vi "vission comm test.vi"() -> ()   [LabVIEW 2009]
uses:
  vision decoder state typedef.ctl
  behaviors/driveable path/drivable paths global.vi
  behaviors/line driveable paths global.vi
  <vilib>/rvi/DataTransferAndStorage/Container/XNode/niFpgaContainer.xnode
  <vilib>/rvi/FIFO/Fifo_Resource/nirvififoUniquifyingName.vi
panel:
  out "x data":i16
  out "y data":i16
  out "DMA timeout":bool
  out "driveable path lengths":u16[](array[numeric])
  out "decoder state":T1
  out "scan number":u8
  in  "allowed proximity squared":i16=100
  in  "Invert Polarity?":bool
  out "driveable path lengths (lines)":u16[](array[numeric])
  out "line  raw serial port data":u8
  out "Number of Elements to Read":u32
  in  "baud rate (9600)":u32=9600
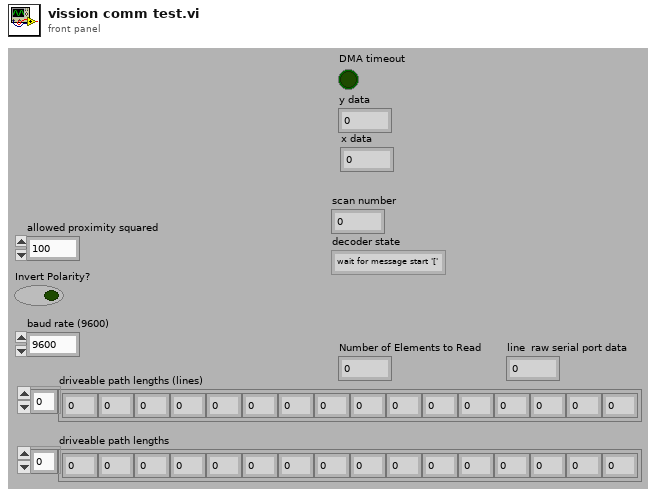
[diagram p1: front panel]
types:
  T1 = typedef "vision decoder state typedef.ctl" = enum16{"wait for message start '['", "wait for point start '(' ", "record x value", "record y value", "scan complete"}
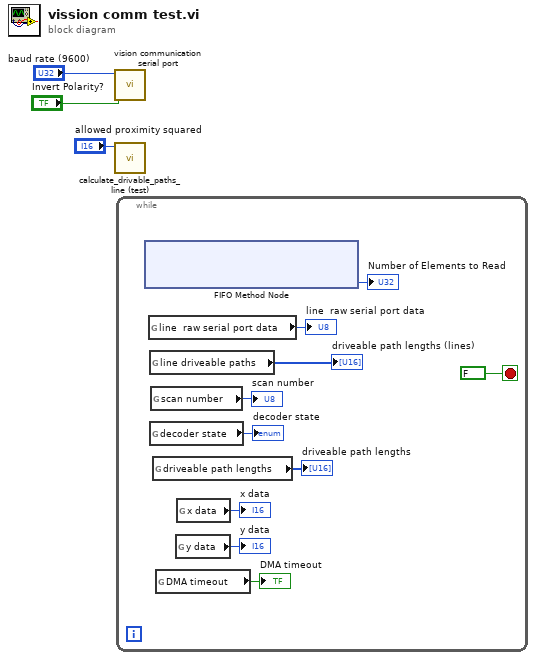
[diagram p0: block diagram]
diagram:
  n1 = call "vision communication serial port.vi"("Invert Polarity?"="Invert Polarity?", "baud rate (9600)"="baud rate (9600)") -> ()  [unwired: 10 in]
  n2 = call "calculate_drivable_paths_line (test).vi"("allowed proximity squared"="allowed proximity squared") -> ()  [unwired: 11 in]
  n3 = while {
    stop <- FALSE stop-if-true
    n4 = xnode ("FIFO Method Node")() -> ("Number of Elements to Read"=→"Number of Elements to Read":u32)  [unwired: 1 in, 1 out]
    n5 = global read "drivable paths global.vi" "line  raw serial port data"() -> (→"line  raw serial port data":u8)
    n6 = global read "line driveable paths global.vi" "line driveable paths"() -> (→"driveable path lengths (lines)":u16[])
    n7 = global read "line driveable paths global.vi" "decoder state"() -> (→"decoder state":T1)
    n8 = global read "line driveable paths global.vi" "scan number"() -> (→"scan number":u8)
    n9 = global read "drivable paths global.vi" "driveable path lengths"() -> (→"driveable path lengths":u16[])
    n10 = global read "line driveable paths global.vi" "DMA timeout"() -> (→"DMA timeout":bool)
    n11 = global read "line driveable paths global.vi" "y data"() -> (→"y data":i16)
    n12 = global read "line driveable paths global.vi" "x data"() -> (→"x data":i16)
  }
